vi "SerialMonitor.vi"() -> ()   [LabVIEW 2014]
uses:
  <vilib>/Instr/_visa.llb/VISA Configure Serial Port (Instr).vi
panel:
  in  "Stop":bool
  in  "Serial Settings":T1={"baud rate"=9600, "data bits"=8, "parity"=enum."None", "stop bits"=10, "flow control"=0} {"flow control" items=["None"=0, "XON/XOFF"=1, "RTS/CTS"=2, "DTR/DSR"=4]; "stop bits" items=["1.0"=10, "1.5"=15, "2.0"=20]; "data bits" min=5 max=8 step=1; "baud rate" items=["75"=75, "110"=110, "134"=134, "150"=150, "300"=300, "600"=600, "1200"=1200, "1800"=1800, "2400"=2400, "4800"=4800, "7200"=7200, "9600"=9600, "14400"=14400, "19200"=19200, "28800"=28800, "38400"=38400, "56000"=56000, "57600"=57600, "115200"=115200, "128000"=128000, "230400"=230400]}
  in  "VISA resource name":refnum<visa-resource-name>="/dev/ttyACM0"
  out "count":i32
  out "Message received":string
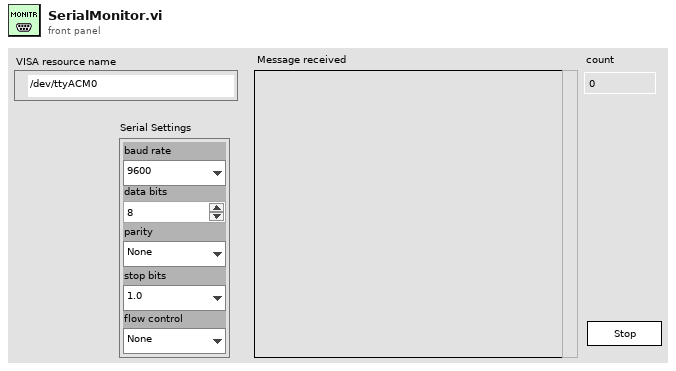
[diagram p1: front panel]
types:
  T1 = cluster{"baud rate":u32, "data bits":u16, "parity":enum16{"None", "Odd", "Even", "Mark", "Space"}, "stop bits":u16, "flow control":u16}
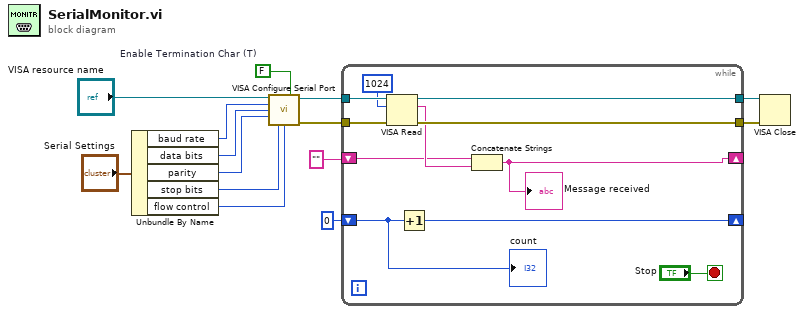
[diagram p0: block diagram]
diagram:
  w1 = FALSE  # Enable Termination Char (T)
  n1 = Unbundle By Name("Serial Settings") -> ("baud rate"=w9:u32, "data bits"=w8:u16, "parity"=w7:enum16{"None", "Odd", "Even", "Mark", "Space"}, "stop bits"=w6:u16, "flow control"=w5:u16)
  n2 = call-poly "VISA Configure Serial Port"("VISA resource name"="VISA resource name", "Enable Termination\nChar (T)"=w1, "baud rate (9600)"=w9, "data bits (8)"=w8, "parity (0:none)"=w7, "stop bits (10: 1 bit)"=w6, "flow control (0:none)"=w5) -> ("VISA resource name out"=w13:refnum<visa-resource-name>, "error out"=w4:errorcluster)  [unwired: 7 in]
  n3 = while {
    shift-right: [w25] -> _
    shift-left: 0 -> [w24]
    tunnel: w13 -> [w23]
    tunnel: [w22] -> w12
    tunnel: w4 -> [w20]
    tunnel: [w19] -> w3
    shift-right: [w15] -> _
    shift-left: "" ("trimmed string") -> [w16]
    stop <- "Stop" stop-if-true
    n4 = VISA Read(VISA resource name=w23, byte count=u32 1024, error in (no error)=w20) -> (VISA resource name out=w22:refnum<visa-resource-name>, read buffer=w17:string, error out=w19:errorcluster)  [unwired: 1 out]
    n5 = Increment(x=w24) -> (x+1=w25:i32)
    n6 = Concatenate Strings(w16, w17) -> (w15:string)
    "Message received" <- w15
    "count" <- w24
  }
  n7 = VISA Close(VISA resource name=w12, error in (no error)=w3) -> ()  [unwired: 1 out]
